vi "IR_OPO_Capture.vi"(0 "GPIB Mode":i16, 1 "STOP CAPTURE":bool, 3 "Y":string="5", 4 "Delay":dbl format="%#_13g", 5 "ESP Port":u8=8, 6 "Delay In":u16, 7 "Axis Speed":string, 9 "Status In":i32, 10 "Commands array":string[][](array[string]), 11 "Laser on/off array 2":bool[][](array[boolean]), 12 "AD status":bool=TRUE, 13 "X":string="5", 14 "error out":errorcluster, 15 "Time array 2":dbl[][](array[numeric])) -> ()   [LabVIEW 2015]
panel:
  out "Capturing":bool
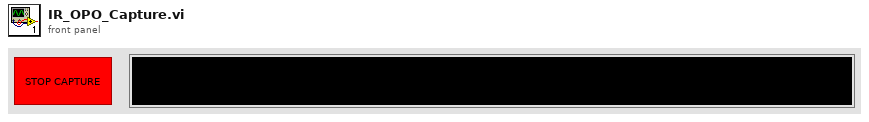
[diagram p1: front panel]
types:
  T1 = enum16{"Initialize", "Lamp ON", "Lamp OFF", "Q-switch ON", "Q-switch OFF", "Adjust Energy", "Change Rep. Rate", "Send String"}
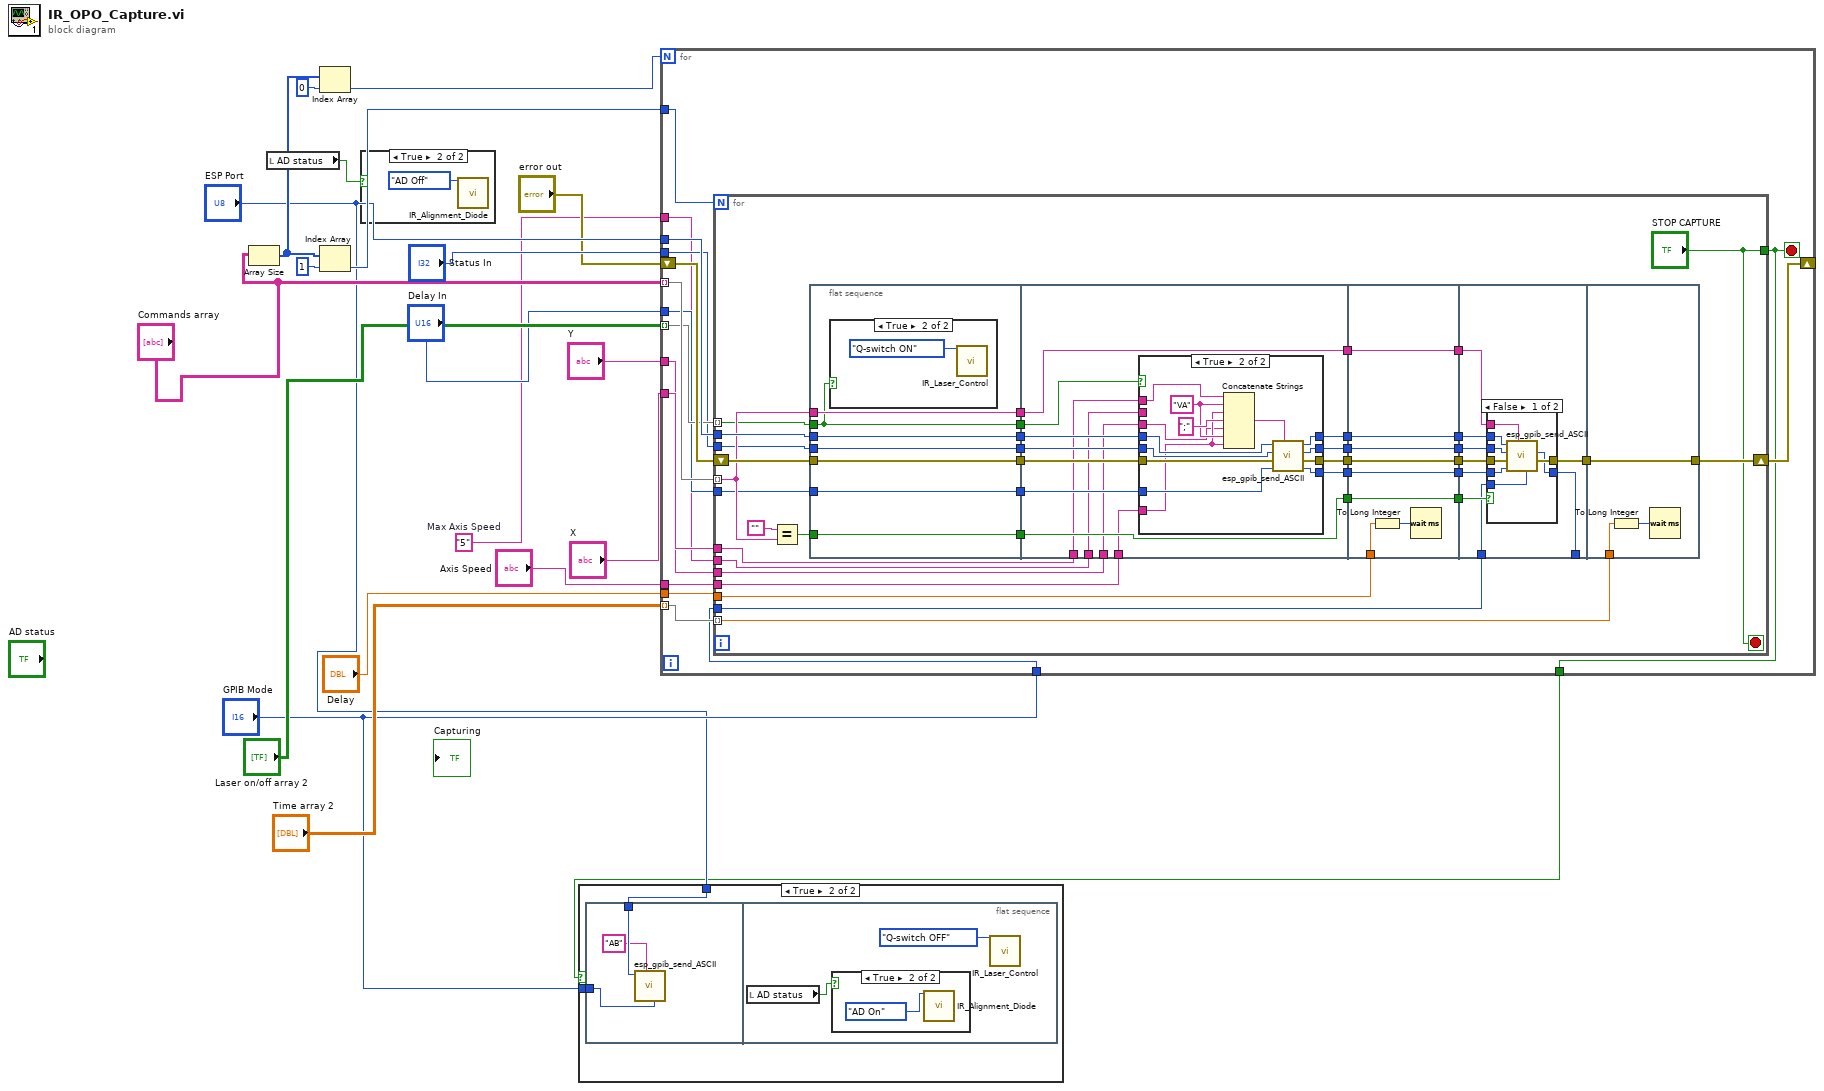
[diagram p0: block diagram]
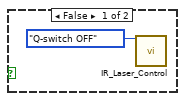
[diagram p3: hidden frame]
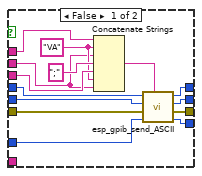
[diagram p4: hidden frame]
diagram:
  w3 = "5"  # Max Axis Speed
  n1 = Array Size(array="Commands array") -> (size(s)=w18:i32[])
  n2 = local read "AD status"() -> (w5:bool)
  n3 = Index Array(array=w18, index=0) -> (element=w19:i32)
  n4 = Index Array(array=w18, index=1) -> (element=w16:i32)
  n5 = case shown="True" w5 {
    frame False {
    }
    frame True {
      n6 = call "IR_Alignment_Diode.vi"("AD Action"=enum16{"AD Off", "AD On"}."AD Off") -> ()  [unwired: 14 in, 1 out]
    }
  }
  n7 = for {
    N: w19 -> [_]
    tunnel: w16 -> [w37]
    tunnel: "Commands array" -> [w36] mode=indexing
    tunnel: "ESP Port" -> [w35]
    shift-right: [w33] -> _
    shift-left: "error out" -> [w34]
    tunnel: "Time array 2" -> [w32] mode=indexing
    tunnel: "Laser on/off array 2" -> [w31] mode=indexing
    tunnel: "Delay" -> [w30]
    tunnel: "GPIB Mode" -> [w29]
    tunnel: [w28] -> w9
    tunnel: "Delay In" -> [w26]
    tunnel: "Status In" -> [w27]
    tunnel: "X" -> [w25]
    tunnel: w3 -> [w24]
    tunnel: "Y" -> [w23]
    tunnel: "Axis Speed" -> [w22]
    stop <- w28 stop-if-true
    n8 = for {
      N: w37 -> [_]
      tunnel: w36 -> [w68] mode=indexing
      tunnel: w35 -> [w74]
      shift-right: [w72] -> w33
      shift-left: w34 -> [w73]
      tunnel: w32 -> [w70] mode=indexing
      tunnel: w31 -> [w63] mode=indexing
      tunnel: w30 -> [w56]
      tunnel: w29 -> [w69]
      tunnel: ["STOP CAPTURE"] -> w28
      tunnel: w26 -> [w64]
      tunnel: w27 -> [w65]
      tunnel: w25 -> [w41]
      tunnel: w24 -> [w40]
      tunnel: w23 -> [w39]
      tunnel: w22 -> [w38]
      stop <- "STOP CAPTURE" stop-if-true
      n9 = Equal?(x="", y=w68) -> (x = y?=w71:bool)
      n10 = flat-sequence {
        tunnel: w64 -> [w76]
        tunnel: w65 -> [w77]
        tunnel: w71 -> [w78]
        tunnel: w73 -> [w79]
        tunnel: w74 -> [w80]
        tunnel: w68 -> [w81]
        tunnel: [w81] -> w54
        tunnel: [w80] -> w52
        tunnel: [w79] -> w50
        tunnel: [w78] -> w48
        tunnel: [w77] -> w46
        tunnel: [w76] -> w45
        tunnel: w63 -> [w75]
        tunnel: [w75] -> w43
        tunnel: w54 -> [w97]
        tunnel: [w97] -> w53
        tunnel: w52 -> [w96]
        tunnel: [w95] -> w51
        tunnel: w50 -> [w91]
        tunnel: [w90] -> w49
        tunnel: w48 -> [w98]
        tunnel: [w98] -> w47
        tunnel: w46 -> [w94]
        tunnel: w45 -> [w89]
        tunnel: [w93] -> w44
        tunnel: w43 -> [w92]
        tunnel: [w88] -> w42
        tunnel: w41 -> [w87]
        tunnel: w40 -> [w86]
        tunnel: w39 -> [w85]
        tunnel: w38 -> [w84]
        tunnel: w53 -> [w134]
        tunnel: [w134] -> w62
        tunnel: w51 -> [w133]
        tunnel: [w133] -> w61
        tunnel: w49 -> [w132]
        tunnel: [w132] -> w60
        tunnel: w47 -> [w131]
        tunnel: [w131] -> w59
        tunnel: [w130] -> w58
        tunnel: [w129] -> w57
        tunnel: w56 -> [w127]
        tunnel: w44 -> [w130]
        tunnel: w42 -> [w129]
        tunnel: [w140] -> w55
        tunnel: w69 -> [w138]
        tunnel: [w136] -> _
        tunnel: w62 -> [w143]
        tunnel: w61 -> [w142]
        tunnel: w60 -> [w141]
        tunnel: w59 -> [w139]
        tunnel: w58 -> [w137]
        tunnel: w57 -> [w135]
        tunnel: w55 -> [w156]
        tunnel: w70 -> [w154]
        tunnel: [w156] -> w72
        frame #0 {
          n11 = case shown="True" w75 {
            frame False {
              n12 = call "IR_Laser_Control.vi"("Action"=T1."Q-switch OFF") -> ()  [unwired: 14 in, 1 out]
            }
            frame True {
              n13 = call "IR_Laser_Control.vi"("Action"=T1."Q-switch ON") -> ()  [unwired: 14 in, 1 out]
            }
          }
        }
        frame #1 {
          n14 = case shown="True" w92 {
            tunnel: [w112 w120] -> w90
            tunnel: w96 -> [w111 w123]
            tunnel: [w110 w118] -> w95
            tunnel: w94 -> [w109 w122]
            tunnel: [w108 w119] -> w93
            tunnel: w91 -> [w107 w121]
            tunnel: w89 -> [w106 w116]
            tunnel: [w105 w117] -> w88
            tunnel: w87 -> [w104 w115]
            tunnel: w86 -> [w99 _]
            tunnel: w85 -> [w101 w113]
            tunnel: w84 -> [_ w114]
            frame False {
              w100 = "VA" ("string")
              n15 = Concatenate Strings(w104, w100, w99, ";" ("string"), w101, w100, w99) -> (w102:string)
              n16 = call "esp_gpib_send_ASCII.vi"("ASCII Cmd"=w102, "Delay In"=w106, "error in"=w107, "Status In"=w109, "Port In"=w111) -> ("Delay Out"=w105:u16, "error out"=w112:errorcluster, "Status Out"=w108:i32, "Port Out"=w110:i32)  [unwired: 2 in, 1 out]
            }
            frame True {
              w124 = "VA" ("string")
              n17 = Concatenate Strings(w115, w124, w114, ";" ("string"), w113, w124, w114) -> (w125:string)
              n18 = call "esp_gpib_send_ASCII.vi"("ASCII Cmd"=w125, "Delay In"=w116, "error in"=w121, "Status In"=w122, "Port In"=w123) -> ("Delay Out"=w117:u16, "error out"=w120:errorcluster, "Status Out"=w119:i32, "Port Out"=w118:i32)  [unwired: 2 in, 1 out]
            }
          }
        }
        frame #2 {
          n19 = To Long Integer(number=w127) -> (32bit integer=w128:i32)
          n20 = Wait (ms)(milliseconds to wait=w128) -> ()  [unwired: 1 out]
        }
        frame #3 {
          n21 = case shown="False" w139 {
            tunnel: w143 -> [w147 _]
            tunnel: w142 -> [w148 _]
            tunnel: w141 -> [w149 w153]
            tunnel: [w150 w153] -> w140
            tunnel: w138 -> [w151 _]
            tunnel: w137 -> [w146 w152]
            tunnel: [w145 w152] -> w136
            tunnel: w135 -> [w144 _]
            frame False {
              n22 = call "esp_gpib_send_ASCII.vi"("mode (0)"=w151, "ASCII Cmd"=w147, "Delay In"=w144, "error in"=w149, "Status In"=w146, "Port In"=w148) -> ("error out"=w150:errorcluster, "Status Out"=w145:i32)  [unwired: 1 in, 3 out]
            }
            frame True {
            }
          }
        }
        frame #4 {
          n23 = To Long Integer(number=w154) -> (32bit integer=w155:i32)
          n24 = Wait (ms)(milliseconds to wait=w155) -> ()  [unwired: 1 out]
        }
      }
    }
  }
  n25 = case shown="True" w9 {
    tunnel: "GPIB Mode" -> [_ w158]
    tunnel: "ESP Port" -> [_ w157]
    frame False {
    }
    frame True {
      n26 = flat-sequence {
        tunnel: w158 -> [w161]
        tunnel: w157 -> [w160]
        frame #0 {
          n27 = call "esp_gpib_send_ASCII.vi"("mode (0)"=w161, "ASCII Cmd"="AB", "Port In"=w160) -> ()  [unwired: 4 in, 5 out]
        }
        frame #1 {
          n28 = local read "AD status"() -> (w162:bool)
          n29 = case shown="True" w162 {
            frame False {
            }
            frame True {
              n30 = call "IR_Alignment_Diode.vi"("AD Action"=enum16{"AD Off", "AD On"}."AD On") -> ()  [unwired: 14 in, 1 out]
            }
          }
          n31 = call "IR_Laser_Control.vi"("Action"=T1."Q-switch OFF") -> ()  [unwired: 14 in, 1 out]
        }
      }
    }
  }
